vi "Endpoint Connected.vi"(8 "error in (no error)":errorcluster, 10 "Endpoint":refnum<class "Message Enqueuer.lvclass">, 11 "Lock-In Remote Actor in":refnum<class "Lock-In Remote Actor.lvclass">) -> (0 "error out":errorcluster, 3 "Lock-In Remote Actor out":refnum<class "Lock-In Remote Actor.lvclass">)   [LabVIEW 2023, in "Lock-In Remote Actor.lvlib" / "Lock-In Remote Actor.lvclass"]
doc: "Override this method to specify how the receiving actor responds to a Connected message from a nested endpoint actor."
uses:
  Lock-In Remote Actor.lvclass
  <vilib>/ActorFramework/Message Enqueuer/Message Enqueuer.lvclass
  Lock-In Remote Actor.lvclass/Lock-In Remote Actor.ctl
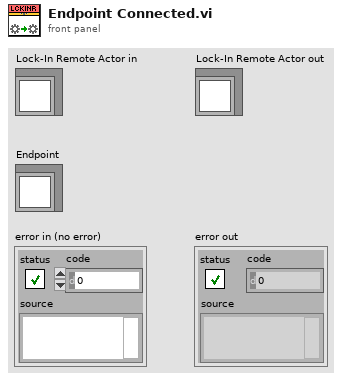
[diagram p1: front panel]
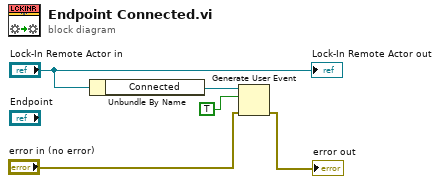
[diagram p0: block diagram]
diagram:
  n1 = Unbundle By Name("Lock-In Remote Actor in") -> ("Connected"=w4:refnum<user-event>)
  n2 = Generate User Event(user event=w4, event data cluster=TRUE ("event data"), error in="error in (no error)") -> (error out=→"error out":errorcluster)  [unwired: 1 in, 1 out]
  "Lock-In Remote Actor out" <- "Lock-In Remote Actor in"
